vi "SubVI_xRecursion.vi"(7 "Enum":T1(ring), 9 "ItemTag":string, 11 "ItemName":string) -> (1 "ItemTags 2":string[](array[string]), 2 "Ident 2":i32[](array[numeric]), 3 "ItemNames 2":string[](array[string]), 4 "FirstAcquired":bool)   [LabVIEW 2016, in "Folder_Mgmt.lvclass"]
uses:
  Folder_Mgmt.lvclass
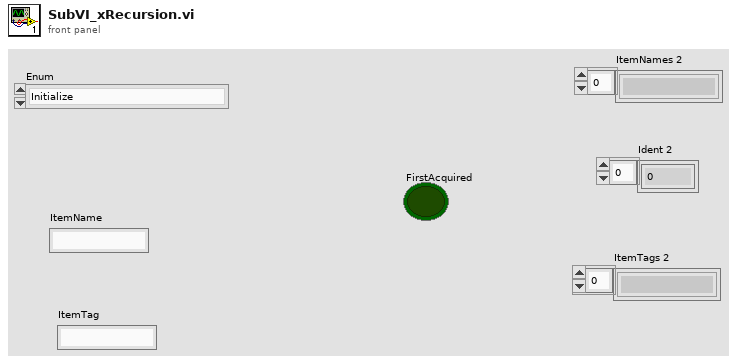
[diagram p1: front panel]
types:
  T1 = enum16{"Initialize", "Get All", "Add ItemName", "Add Ident", "Add Item Tag", "CurrIdentPlus", "CurrIdentMinus", "ResetFirstAcquired"}
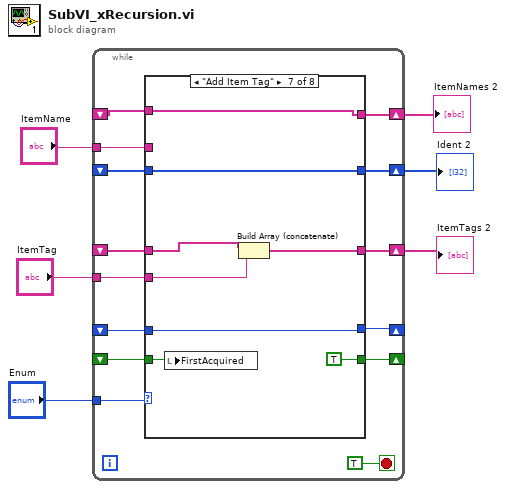
[diagram p0: block diagram]
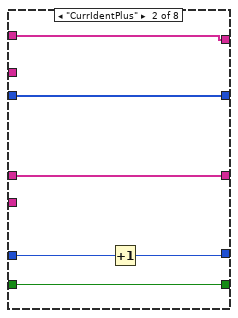
[diagram p3: hidden frame]
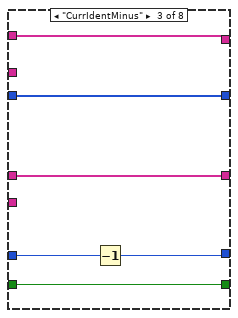
[diagram p4: hidden frame]
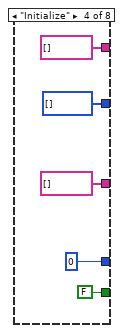
[diagram p5: hidden frame]
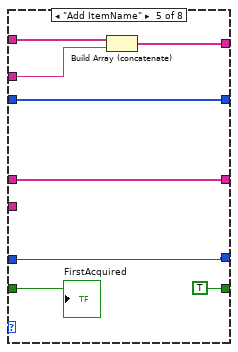
[diagram p6: hidden frame]
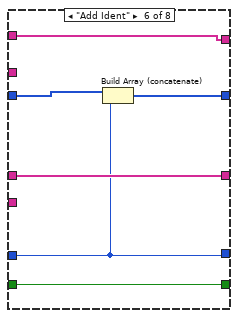
[diagram p7: hidden frame]
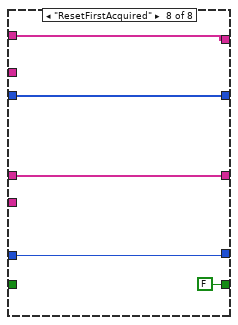
[diagram p8: hidden frame]
diagram:
  n1 = while {
    tunnel: "Enum" -> [w19]
    tunnel: "ItemName" -> [w18]
    shift-right: [w17] -> w3
    shift-left: _ -> [w16]
    shift-right: [w15] -> w2
    shift-left: _ -> [w14]
    tunnel: "ItemTag" -> [w13]
    shift-right: [w12] -> w1
    shift-left: _ -> [w11]
    shift-right: [w10] -> _
    shift-left: _ -> [w9]
    shift-right: [w8] -> _
    shift-left: _ -> [w7]
    stop <- TRUE stop-if-true
    n2 = case shown="\"Add Item Tag\"" w19 {
      tunnel: w18 -> [_ _ _ _ w50 _ _ _]
      tunnel: [w25 w29 w35 string[] [] w49 w54 w64 w69] -> w17
      tunnel: w16 -> [w25 w29 w35 _ w48 w54 w64 w69]
      tunnel: [w24 w28 w34 i32[] [] w47 w56 w60 w68] -> w15
      tunnel: w14 -> [w24 w28 w34 _ w47 w55 w60 w68]
      tunnel: w13 -> [_ _ _ _ _ _ w63 _]
      tunnel: [w23 w27 w33 string[] [] w46 w53 w62 w67] -> w12
      tunnel: w11 -> [w23 w27 w33 _ w46 w53 w61 w67]
      tunnel: [w22 w30 w36 0 w45 w52 w59 w66] -> w10
      tunnel: w9 -> [w22 w31 w37 _ w45 w52 w59 w66]
      tunnel: [w21 w26 w32 FALSE TRUE w51 TRUE FALSE] -> w8
      tunnel: w7 -> [w21 w26 w32 _ w43 w51 w57 _]
      frame "Get All", Default {
      }
      frame "CurrIdentPlus" {
        n3 = Increment(x=w31) -> (x+1=w30:i32)
      }
      frame "CurrIdentMinus" {
        n4 = Decrement(x=w37) -> (x-1=w36:i32)
      }
      frame "Initialize" {
      }
      frame "Add ItemName" {
        n5 = Build Array (concatenate)(w48, w50) -> (w49:string[])
        "FirstAcquired" <- w43
      }
      frame "Add Ident" {
        n6 = Build Array (concatenate)(w55, w52) -> (w56:i32[])
      }
      frame "Add Item Tag" {
        n7 = local write "FirstAcquired"(w57) -> ()
        n8 = Build Array (concatenate)(w61, w63) -> (w62:string[])
      }
      frame "ResetFirstAcquired" {
      }
    }
  }
  "ItemNames 2" <- w3
  "Ident 2" <- w2
  "ItemTags 2" <- w1
